vi "Big_Temporal.vi"(3 "Feature Selection":u16, 4 "Session Index":i32, 5 "Experment Index":i32, 6 "Array in":dbl[][](array[numeric])) -> (0 "Ending Frequency\nin Wave (Hz)":dbl, 1 "Starting Frequency\nin Wave (Hz)":dbl, 2 "Dominant Frequency\nin Wave (Hz)":dbl)   [LabVIEW 2023]
panel:
  in  "Frequency Saver?":bool=TRUE
  in  "Threshold\nPercentage":dbl=0.05
  in  "FFT Size":i32=10000000
  in  "Normalize\nData":bool
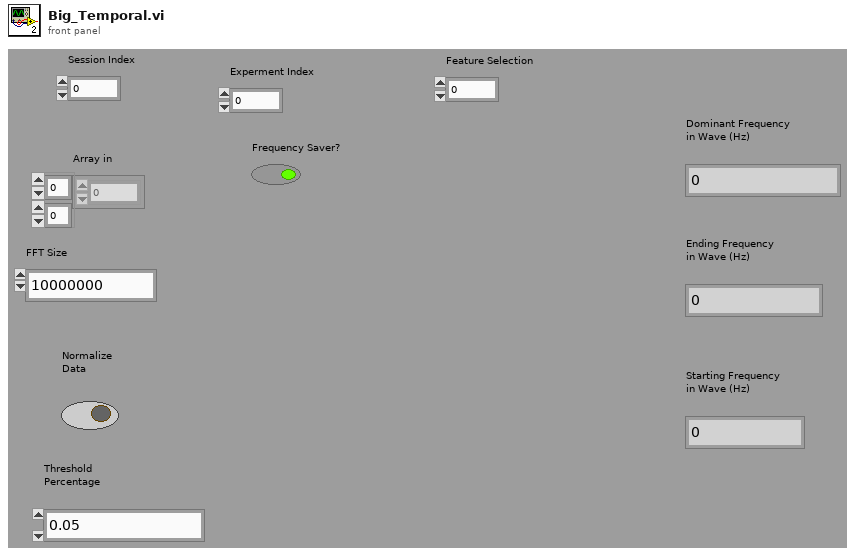
[diagram p1: front panel]
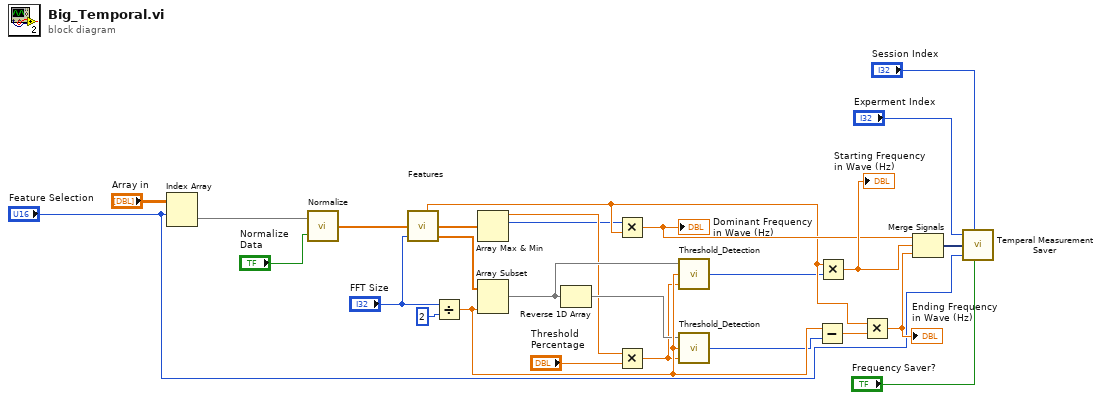
[diagram p0: block diagram]
diagram:
  n1 = Index Array "Index Array"(array="Array in", index (row)="Feature Selection") -> (element=w7:dbl[])  [unwired: 1 in]
  n2 = call "Normalize.vi"("Normalize Data"="Normalize\nData", "Array in"=w7) -> ("Array out"=w10:dbl[])
  n3 = call "Features.vi"("Array in"=w10, "Sampling"="FFT Size") -> ("Frequency Resolution"=w24:dbl, "FFT"=w8:dbl[], "abs(FFT)"=w12:dbl[])  [unwired: 3 in, 2 out]
  n4 = Divide(x="FFT Size", y=2) -> (x/y=w21:dbl)
  n5 = Array Max & Min(array=w8) -> (max value=w16:dbl, max index (indices)=w11:i32)  [unwired: 2 out]
  n6 = Array Subset "Array Subset"(array=w12, length=w21) -> (w19:dbl[])  [unwired: 1 in]
  n7 = Reverse 1D Array(array=w19) -> (reversed array=w18:dbl[])
  n8 = Multiply(x=w11, y=w24) -> (x*y=w25:dbl)
  "Dominant Frequency\nin Wave (Hz)" <- w25
  n9 = Multiply(x=w16, y="Threshold\nPercentage") -> (x*y=w17:dbl)
  n10 = call "Threshold_Detection.vi"("Threshold Value"=w17, "Length of Array"=w21, "Array"=w19) -> ("Detection Index"=w22:i32)
  n11 = call "Threshold_Detection.vi"("Threshold Value"=w17, "Length of Array"=w21, "Array"=w18) -> ("Detection Index"=w20:i32)
  n12 = Subtract(x=w21, y=w20) -> (x-y=w23:dbl)
  n13 = Multiply(x=w24, y=w22) -> (x*y=w26:dbl)
  "Starting Frequency\nin Wave (Hz)" <- w26
  n14 = Multiply(x=w24, y=w23) -> (x*y=w27:dbl)
  "Ending Frequency\nin Wave (Hz)" <- w27
  n15 = Merge Signals(w25, w26, w27) -> (w3:dynamicdata)
  n16 = call "Temperal Measurement Saver.vi"("Experiment Index"="Experment Index", "Session Index"="Session Index", "Dynamic Data"=w3, "Feature Index"="Feature Selection", "Frequency Saver?"="Frequency Saver?") -> ()  [unwired: 1 in]
